vi "SetParam.vi"(8 "error in (no error)":errorcluster caption="entrée d'erreur (pas d'erreur)", 10 "classification_report":T1={"labels"=[], "target_names"=[], "sample_weight"=[], "digits"=2, "zero_division"={"dtype_zero_division"="str", "zero_division"="warn"}}, 11 "Classification_Report.lvclass":refnum<class "Classification_Report.lvclass">) -> (0 "error out":errorcluster caption="sortie d'erreur", 3 "Classification_Report.lvclass":refnum<class "Classification_Report.lvclass">)   [LabVIEW 2020, in "Classification_Report.lvclass"]
doc: "Set Parameters"
uses:
  Classification_Report.lvclass
  Classification_Report.lvclass/Classification_Report.ctl
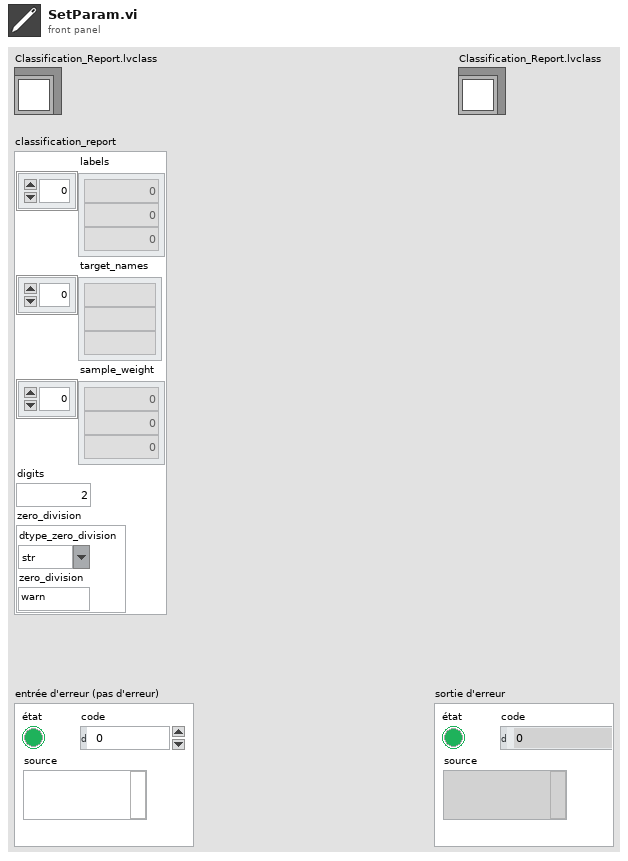
[diagram p1: front panel]
types:
  T1 = cluster{"labels":i32[], "target_names":string[], "sample_weight":dbl[], "digits":i32, "zero_division":cluster{"dtype_zero_division":string, "zero_division":string}}
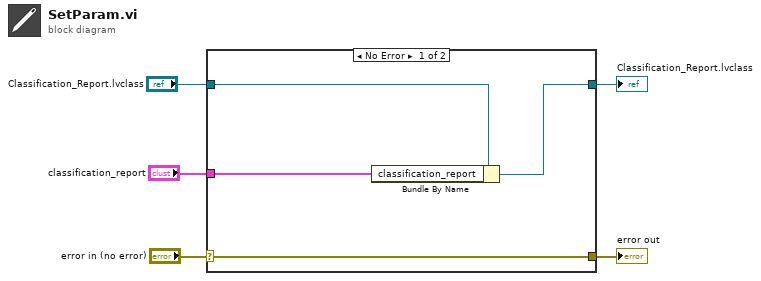
[diagram p0: block diagram]
diagram:
  n1 = case shown="No Error" "error in (no error)" {
    selector: "error in (no error)" -> [w9 w10]
    tunnel: [w9 w10] -> w4
    tunnel: [w7 w11] -> w2
    tunnel: "Classification_Report.lvclass" -> [w8 w11]
    tunnel: "classification_report" -> [w6 _]
    frame No Error {
      n2 = Bundle By Name(cluster=w8, "classification_report"=w6) -> (w7:refnum<class "Classification_Report.lvclass">)
    }
    frame Error {
    }
  }
  "error out" <- w4
  "Classification_Report.lvclass" <- w2
